vi "Fault Handling.vi"(8 "error in (no error)":errorcluster, 10 "FaultCode":i32, 11 "OPC UA in":refnum<class "OPC UA.lvclass">) -> (0 "error out":errorcluster, 3 "OPC UA out":refnum<class "OPC UA.lvclass">)   [LabVIEW 2021, in "OPC UA.lvclass"]
uses:
  OPC UA.lvclass
  OPC UA.lvclass/OPC UA.ctl
panel:
  out "Fault":bool
  out "Description":string
  out "Fault Bits":bool[](array[boolean])
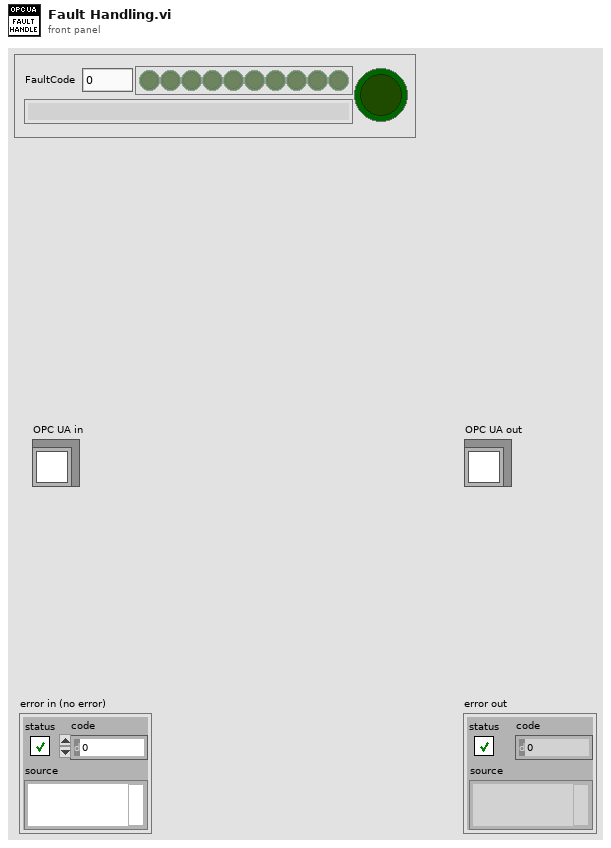
[diagram p1: front panel]
types:
  T1 = enum32{"Invalid", "Standard", "Closed", "Hidden", "Minimized", "Maximized"}
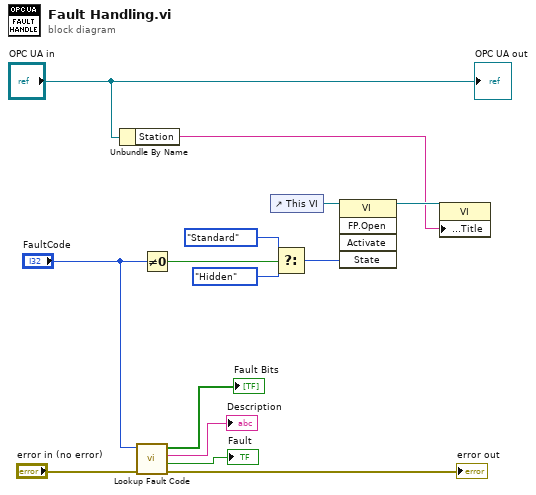
[diagram p0: block diagram]
diagram:
  n1 = Unbundle By Name("OPC UA in") -> ("Station"=w1:string)
  n2 = call "Lookup Fault Code.vi"("error in (no error)"="error in (no error)", "FaultCode"="FaultCode") -> ("error out"=→"error out":errorcluster, "Fault"=→"Fault":bool, "Description"=→"Description":string, "Fault Bits"=→"Fault Bits":bool[])  [unwired: 6 in]
  n3 = Not Equal To 0?(x="FaultCode") -> (x != 0?=w9:bool)
  n4 = control-ref of="This VI"() -> (w4:refnum<vi>)
  n5 = Select(t=T1."Standard" ("State"), s=w9, f=T1."Hidden" ("State")) -> (s? t:f=w6:T1)
  n6 = invoke class="VI" method="FP.Open"(reference=w4, "State"=w6) -> (reference out=w5:refnum<vi>)  [unwired: 3 in, 4 out]
  n7 = property class="VI"(reference=w5, "Front Panel.Title"=w1) -> ()  [unwired: 1 in, 2 out]
  "OPC UA out" <- "OPC UA in"
